vi "ButtonPressedTest.vi"() -> ()   [LabVIEW 2015]
panel:
  out "DoSomething":bool=TRUE
  in  "stop":bool
  out "Button Presses":bool[](array[boolean])
  in  "Button Values":bool[](array[boolean])
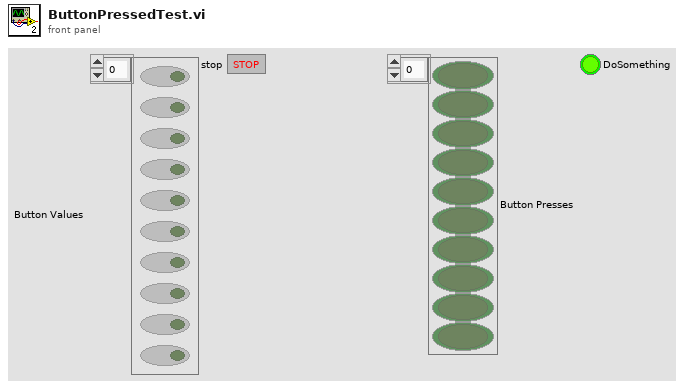
[diagram p1: front panel]
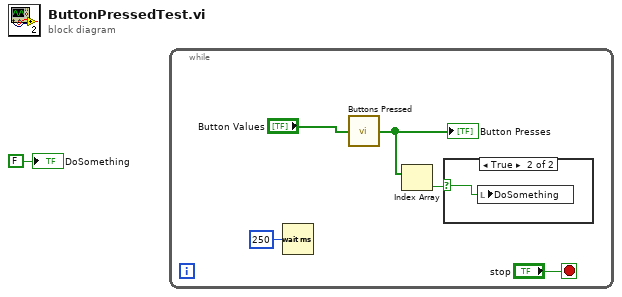
[diagram p0: block diagram]
diagram:
  n1 = while {
    stop <- "stop" stop-if-true
    n2 = Wait (ms)(milliseconds to wait=u32 250) -> ()  [unwired: 1 out]
    n3 = call "Buttons Pressed.vi"("Button Values"="Button Values") -> ("Button Presses"=w3:bool[])
    "Button Presses" <- w3
    n4 = Index Array(array=w3) -> (element=w2:bool)  [unwired: 1 in]
    n5 = case shown="True" w2 {
      selector: w2 -> [_ w7]
      frame False {
      }
      frame True {
        n6 = local write "DoSomething"(w7) -> ()
      }
    }
  }
  "DoSomething" <- FALSE ("DoSomething")
